vi "NIFPGA-MCS.read data.vi"(0 "i ref in":refnum<vi>, 5 "error in (no error)":errorcluster) -> (14 "i ref out":refnum<vi>, 16 "Output Waveform":T1, 19 "error out":errorcluster)   [LabVIEW 2014, in "NIFPGA-MCS.lvlib"]
doc: "(D:1;D:1;D:N) n[t0, dT, data] //performs the sequence StopScan - GetBinData - StartScan. It is the task of the developer to program the internal sequence of commands such, that the device can be used by just sending repeated ReadData commands."
uses:
  NIFPGA-MCS.lvlib
  CSCore/CSSystem/CoreDefs/CoreDefs.rawDataType.ctl
  CSCore/CSApplicationBaseClasses/MCSBase/MCSBase.statusType.ctl
  CSCore/CSApplicationBaseClasses/MCSBase/MCSBase.directionType.ctl
  CSCore/CSApplicationBaseClasses/MCSBase/MCSBase.serviceType.ctl
  CSlibraries/UtilityLib/UtilityLib.valueStatus.ctl
  CSCore/CSSystem/CoreDefs/CoreDefs.error_type.ctl
  CSCore/CSSystem/CoreDefs/CoreDefs.error_severity.ctl
  CSCore/CSApplicationBaseClasses/DeviceBase/DeviceBase.lvlib
  CSCore/CSApplicationBaseClasses/MCSBase/MCSBase.lvlib
  CSlibraries/UtilityLib/UtilityLib.lvlib
  CSCore/CSSystem/CoreLib/CoreLib.lvlib
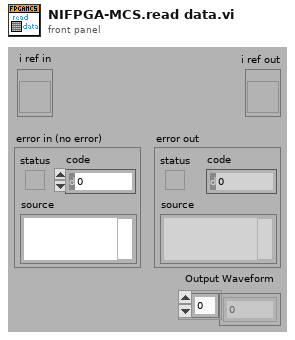
[diagram p1: front panel]
types:
  T1 = typedef "CoreDefs.rawDataType.ctl" = i8[]
  T2 = typedef "UtilityLib.lvlib/UtilityLib.valueStatus.ctl" = enum16{"no info available", "stand by/off", "on", "warning", "alarm/malfunction", "not implemented", "user action required", "important information", "system default", "control default", "indicator default", "button default"}
  T3 = typedef "MCSBase.lvlib/MCSBase.serviceType.ctl" = enum16{"counts", "totalCounts", "binWidth", "nOfBins", "nOfRecords", "status", "discrLevel", "discrSlope", "triggerLevel", "triggerSlope"}
  T4 = typedef "MCSBase.lvlib/MCSBase.directionType.ctl" = enum16{"unknown", "update actual value", "update nominal value", "update both"}
  T5 = typedef "CoreDefs.error_severity.ctl" = enum16{"undefined", "information", "warning", "error", "fatal"}
  T6 = typedef "CoreDefs.error_type.ctl" = enum16{"no error", "can't load process", "can't unload process", "process does not exist", "can't install process", "can't remove process", "unknown function", "time out", "can't execute function", "duplicate queue name", "super not found", "caller queue invalid", "can't ping process", "unknown error", "VISA Error", "VISA timeout", "GPIB timeout", "GPIB error", "communication error", "data type mismatch", "can't read data from OPC server", "can't write data to OPC server", "OET error", "function not implemented", "process already exists", "invalid Shared Variable name", "error writing Shared Variable", "error reading Shared Variable", "invalid client name", "corrupt database", "unknown class", "call not authorized", "parameter out of range", "OET timeout: can't get data to modify", "invalid queue name", "requested operation incompatible with current state", "event undefined", "event disabled", "state undefined", "caller is not a friend", "EventBuilder: bad eventID", "EventBuilder: no DAQ devices", "a thread must not stop itself", "UNUSED ELEMENT4", "DiscArchiver: eventData incomplete", "DiscArchiver: eventData does not belong to run", "DiscArchiver: can't open file", "DiscArchiver: can't write to file", "DiscArchiver: available disc space low", "can't acquire semaphore", "error reading data from database", "notifier object is not existing", "can't register process", "can't unregister process", "illegal event type", "object disabled", "object already exists", "can't change state", "Instrument not found", "no connection to remote node", "invalid reference", "N/A", "UNUSED ELEMENT 1", "element not found", "illegal TCP/IP connection detected", "object does not exist", "invalid access ID", "unknown CS system", "invalid privilige", "unsupported data type", "unsupported server type", "IO server already exists", "Shared Variable already exists"}
  T7 = typedef "MCSBase.lvlib/MCSBase.statusType.ctl" = i32
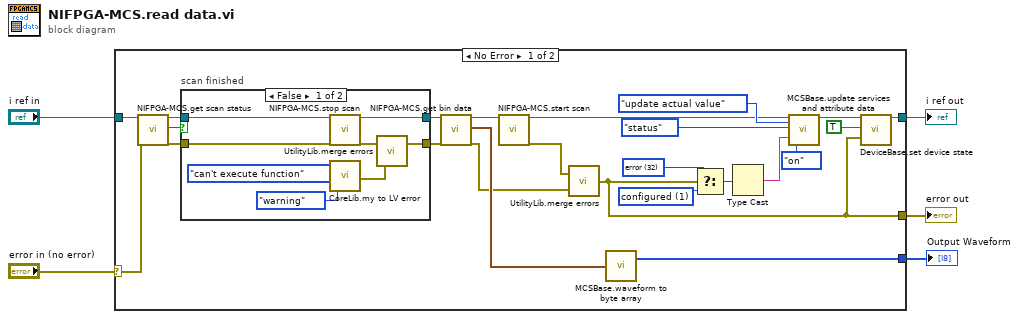
[diagram p0: block diagram]
diagram:
  n1 = case shown="No Error" "error in (no error)" {
    selector: "error in (no error)" -> [w13 w40]
    tunnel: "i ref in" -> [w15 w41]
    tunnel: [w19 w41] -> w3
    tunnel: [w18 w40] -> w2
    tunnel: [w16 _] -> w1
    frame No Error {
      w24 = T7 32 items=["unknown"=0, "configured"=1, "error"=32] ("t")
      w23 = T7 1 items=["unknown"=0, "configured"=1, "error"=32] ("service")
      n2 = call "NIFPGA-MCS.get scan status.vi"("i ref in"=w15, "error in (no error)"=w13) -> ("i ref out"=w11:refnum<vi>, "scanFinished ?"=w12:bool, "error out"=w8:errorcluster)  [unwired: 14 in, 1 out]
      n3 = case "scan finished" shown="False" w12 {
        tunnel: w11 -> [w37 w39]
        tunnel: [w36 w39] -> w10
        tunnel: [w32 w38] -> w9
        tunnel: w8 -> [w33 w38]
        frame False {
          n4 = call "NIFPGA-MCS.stop scan.vi"("i ref in"=w37, "error in (no error)"=w33) -> ("i ref out"=w36:refnum<vi>, "error out"=w31:errorcluster)  [unwired: 15 in, 1 out]
          n5 = call "CoreLib.my to LV error.vi"("ErrorTypes"=CoreDefs.error_type."can't execute function", "severityLevel"=CoreDefs.error_severity."warning") -> ("myErrorCluster"=w30:errorcluster)  [unwired: 16 in, 1 out]
          n6 = call "UtilityLib.merge errors.vi"("error2 (no error)"=w30, "error1 (no error)"=w31) -> ("error out"=w32:errorcluster)
        }
        frame True {
        }
      }
      n7 = call "NIFPGA-MCS.get bin data.vi"("i ref in"=w10, "error in (no error)"=w9) -> ("i ref out"=w14:refnum<vi>, "Output Waveform"=w17:waveform(dbl), "error out"=w6:errorcluster)  [unwired: 15 in]
      n8 = call "NIFPGA-MCS.start scan.vi"("i ref in"=w14) -> ("i ref out"=w20:refnum<vi>, "error out"=w7:errorcluster)  [unwired: 16 in, 1 out]
      n9 = call "UtilityLib.merge errors.vi"("error2 (no error)"=w6, "error1 (no error)"=w7) -> ("error out"=w18:errorcluster)
      n10 = call "MCSBase.waveform to byte array.vi"("Waveform"=w17) -> ("byteArray out"=w16:T1)  [unwired: 1 out]
      n11 = Select(t=w24, s=w18, f=w23) -> (s? t:f=w25:T7)
      n12 = Type Cast(x=w25) -> (*(type *) &x=w26:string)  [unwired: 1 in]
      n13 = call "MCSBase.update services and attribute data.vi"("i ref in"=w20, "direction"=MCSBase.directionType."update actual value", "service"=MCSBase.serviceType."status", "value"=w26, "quality"=UtilityLib.valueStatus."on") -> ("i ref out"=w28:refnum<vi>)  [unwired: 12 in, 2 out]
      n14 = call "DeviceBase.set device state.vi"("i ref in"=w28, "implicit"=TRUE, "device error"=w18) -> ("i ref out"=w19:refnum<vi>)  [unwired: 14 in, 2 out]
    }
    frame Error {
    }
  }
  "error out" <- w2
  "i ref out" <- w3
  "Output Waveform" <- w1
